vi "Decode Session Information Packet.vi"(10 "JSONInput":string) -> (2 "sessionInformation":T1)   [LabVIEW 2014]
uses:
  Session Information.ctl
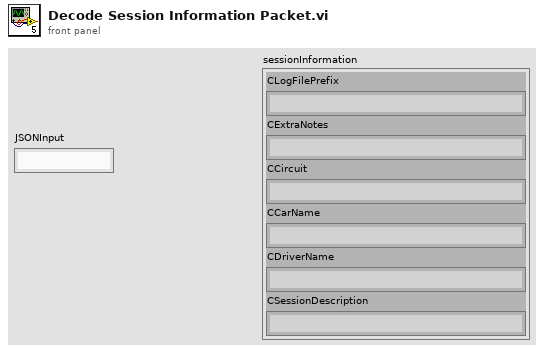
[diagram p1: front panel]
types:
  T1 = typedef "Session Information.ctl" = cluster{"CLogFilePrefix":string, "CExtraNotes":string, "CCircuit":string, "CCarName":string, "CDriverName":string, "CSessionDescription":string}
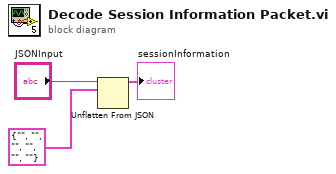
[diagram p0: block diagram]
diagram:
  n1 = Unflatten From JSON(JSON string="JSONInput", type and defaults=T1 {"CLogFilePrefix"="", "CExtraNotes"="", "CCircuit"="", "CCarName"="", "CDriverName"="", "CSessionDescription"=""} ("Session Information")) -> (value=→"sessionInformation":T1)  [unwired: 5 in, 1 out]
